vi "Initialize.vi"(8 "error in (no error)":errorcluster, 10 "DeviceName":string, 11 "HexapodController in":refnum<class "Tapedrive_ESP301.lvclass">) -> (0 "error out":errorcluster, 1 "new command(s)":string, 2 "DeviceName":string, 3 "HexapodController out":refnum<class "Tapedrive_ESP301.lvclass">)   [LabVIEW 2011, in "Tapedrive_ESP301.lvclass"]
uses:
  Tapedrive_ESP301.lvclass
  BaseDriver/BaseDriver.lvclass
  Tapedrive_ESP301.lvclass/Tapedrive_ESP301.ctl
  Newport ESP301.lvlib
panel:
  out "Cleared Error Queue":string
  out "Settings.devport":string
  out "Connected":bool
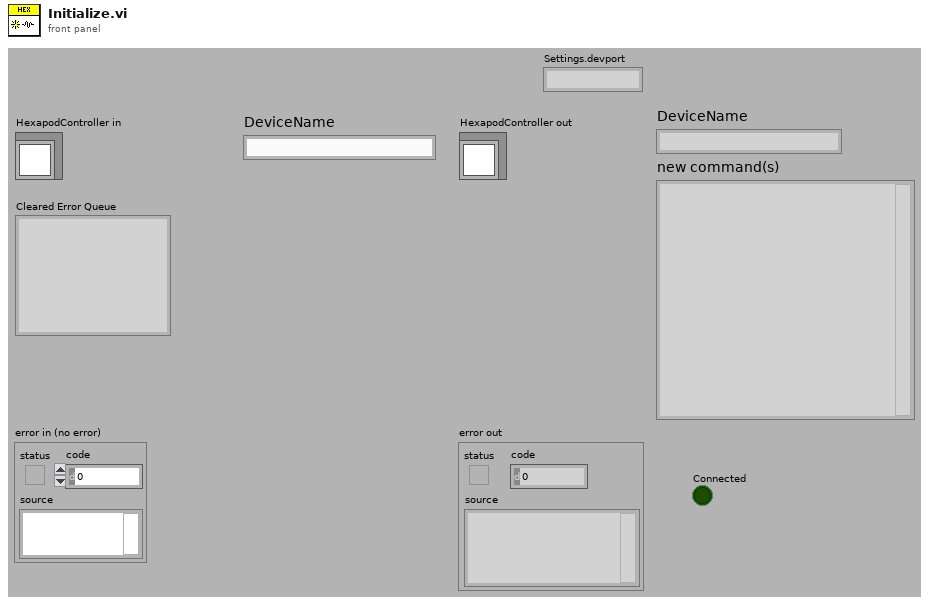
[diagram p1: front panel]
types:
  T1 = typedef "Tapedrive_ESP301.lvclass/settingsCluster_TapeDrive_TypDef.ctl" = cluster{"devport":string, "tapepos":cluster{"Value":dbl, "Min":dbl, "Max":dbl, "StepSize":dbl, "Tolerance":dbl, "ValueActual":dbl}, "status":enum16{"Not referenced", "Homing", "Moving", "Ready"}, "inmotion":T2, "forwardaxis":i16, "backwardaxis":i16, "encoderaxis":i16, "Velocity":cluster{"Axis 1":cluster{"Value":dbl, "Min":dbl, "Max":dbl, "StepSize":dbl, "Tolerance":dbl, "ValueActual":dbl}, "Axis 2":cluster{"Value":dbl, "Min":dbl, "Max":dbl, "StepSize":dbl, "Tolerance":dbl, "ValueActual":dbl}}, "Acceleration":cluster{"Axis 1":cluster{"Value":dbl, "Min":dbl, "Max":dbl, "StepSize":dbl, "Tolerance":dbl, "ValueActual":dbl}, "Axis 2":cluster{"Value":dbl, "Min":dbl, "Max":dbl, "StepSize":dbl, "Tolerance":dbl, "ValueActual":dbl}}, "Decceleration":cluster{"Axis 1":cluster{"Value":dbl, "Min":dbl, "Max":dbl, "StepSize":dbl, "Tolerance":dbl, "ValueActual":dbl}, "Axis 2":cluster{"Value":dbl, "Min":dbl, "Max":dbl, "StepSize":dbl, "Tolerance":dbl, "ValueActual":dbl}}, "MaxAcceleration":cluster{"Axis 1":cluster{"Value":dbl, "Min":dbl, "Max":dbl, "StepSize":dbl, "Tolerance":dbl, "ValueActual":dbl}, "Axis 2":cluster{"Value":dbl, "Min":dbl, "Max":dbl, "StepSize":dbl, "Tolerance":dbl, "ValueActual":dbl}}, "MaxVelocity":cluster{"Axis 1":cluster{"Value":dbl, "Min":dbl, "Max":dbl, "StepSize":dbl, "Tolerance":dbl, "ValueActual":dbl}, "Axis 2":cluster{"Value":dbl, "Min":dbl, "Max":dbl, "StepSize":dbl, "Tolerance":dbl, "ValueActual":dbl}}, "VelocityFFG":cluster{"Axis 1":cluster{"Value":dbl, "Min":dbl, "Max":dbl, "StepSize":dbl, "Tolerance":dbl, "ValueActual":dbl}, "Axis 2":cluster{"Value":dbl, "Min":dbl, "Max":dbl, "StepSize":dbl, "Tolerance":dbl, "ValueActual":dbl}}, "AccelerationFFG":cluster{"Axis 1":cluster{"Value":dbl, "Min":dbl, "Max":dbl, "StepSize":dbl, "Tolerance":dbl, "ValueActual":dbl}, "Axis 2":cluster{"Value":dbl, "Min":dbl, "Max":dbl, "StepSize":dbl, "Tolerance":dbl, "ValueActual":dbl}}, "DACoffset":cluster{"Axis 1":cluster{"Value":dbl, "Min":dbl, "Max":dbl, "StepSize":dbl, "Tolerance":dbl, "ValueActual":dbl}, "Axis 2":cluster{"Value":dbl, "Min":dbl, "Max":dbl, "StepSize":dbl, "Tolerance":dbl, "ValueActual":dbl}}, "Power":cluster{"Axis 1":T2, "Axis 2":T2}, "ReductionRatio":cluster{"Value":dbl, "Min":dbl, "Max":dbl, "StepSize":dbl, "Tolerance":dbl, "ValueActual":dbl}, "Direction":T3, "Tension":T2, "TensionVelocity":cluster{"Axis 1":cluster{"Value":dbl, "Min":dbl, "Max":dbl, "StepSize":dbl, "Tolerance":dbl, "ValueActual":dbl}, "Axis 2":cluster{"Value":dbl, "Min":dbl, "Max":dbl, "StepSize":dbl, "Tolerance":dbl, "ValueActual":dbl}}, "TensionAcceleration":cluster{"Axis 1":cluster{"Value":dbl, "Min":dbl, "Max":dbl, "StepSize":dbl, "Tolerance":dbl, "ValueActual":dbl}, "Axis 2":cluster{"Value":dbl, "Min":dbl, "Max":dbl, "StepSize":dbl, "Tolerance":dbl, "ValueActual":dbl}}, "TensionDecceleration":cluster{"Axis 1":cluster{"Value":dbl, "Min":dbl, "Max":dbl, "StepSize":dbl, "Tolerance":dbl, "ValueActual":dbl}, "Axis 2":cluster{"Value":dbl, "Min":dbl, "Max":dbl, "StepSize":dbl, "Tolerance":dbl, "ValueActual":dbl}}, "MoveVelocity":cluster{"Axis 1":cluster{"Value":dbl, "Min":dbl, "Max":dbl, "StepSize":dbl, "Tolerance":dbl, "ValueActual":dbl}, "Axis 2":cluster{"Value":dbl, "Min":dbl, "Max":dbl, "StepSize":dbl, "Tolerance":dbl, "ValueActual":dbl}}, "MoveAcceleration":cluster{"Axis 1":cluster{"Value":dbl, "Min":dbl, "Max":dbl, "StepSize":dbl, "Tolerance":dbl, "ValueActual":dbl}, "Axis 2":cluster{"Value":dbl, "Min":dbl, "Max":dbl, "StepSize":dbl, "Tolerance":dbl, "ValueActual":dbl}}, "MoveDecceleration":cluster{"Axis 1":cluster{"Value":dbl, "Min":dbl, "Max":dbl, "StepSize":dbl, "Tolerance":dbl, "ValueActual":dbl}, "Axis 2":cluster{"Value":dbl, "Min":dbl, "Max":dbl, "StepSize":dbl, "Tolerance":dbl, "ValueActual":dbl}}, "MaxStepsize":cluster{"Value":dbl, "Min":dbl, "Max":dbl, "StepSize":dbl, "Tolerance":dbl, "ValueActual":dbl}, "Stepsize":cluster{"Value":dbl, "Min":dbl, "Max":dbl, "StepSize":dbl, "Tolerance":dbl, "ValueActual":dbl}, "GoStep":T2, "StopWait":T2, "stepnum":cluster{"Value":dbl, "Min":dbl, "Max":dbl, "StepSize":dbl, "Tolerance":dbl, "ValueActual":dbl}, "MoveIfScan":T2, "HomeEncoder":T2, "Timeout":cluster{"Value":dbl, "Min":dbl, "Max":dbl, "StepSize":dbl, "Tolerance":dbl, "ValueActual":dbl}, "TapeRelax":cluster{"Value":dbl, "Min":dbl, "Max":dbl, "StepSize":dbl, "Tolerance":dbl, "ValueActual":dbl}}
  T2 = typedef "OnOffTypeDef.ctl" = enum16{"off", "on"}
  T3 = typedef "Direction.ctl" = enum16{"Forward", "Backward", "Undefined"}
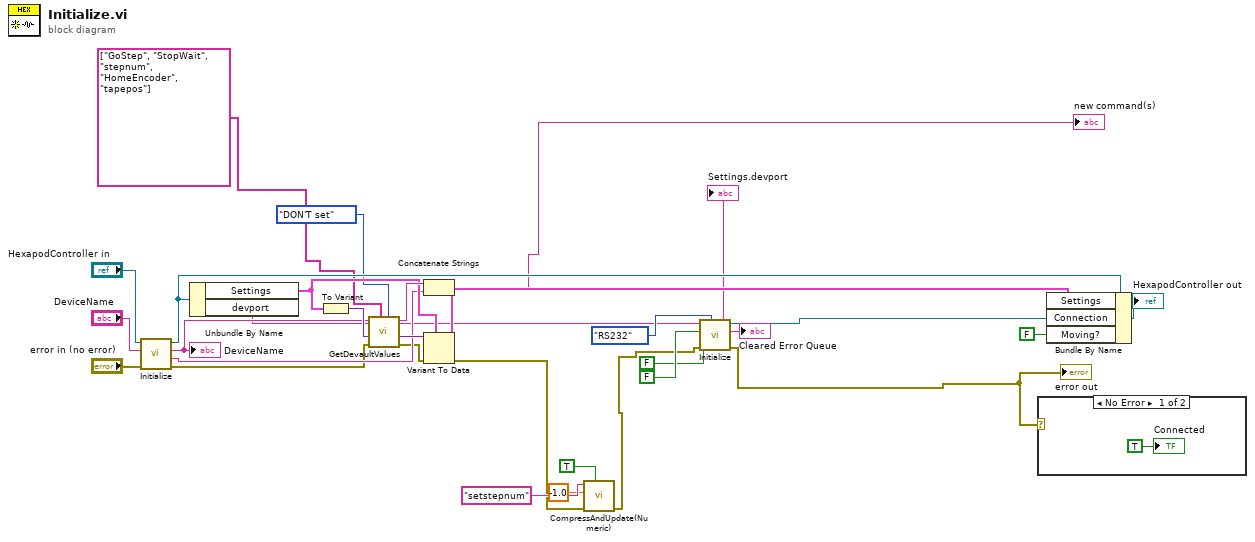
[diagram p0: block diagram]
diagram:
  n1 = call-parent "Initialize.vi"("error in (no error)"="error in (no error)", "DeviceName"="DeviceName", "BaseDriver in"="HexapodController in") -> ("error out"=w17:errorcluster, "new command(s)"=w22:string, "DeviceName"=w23:string, "BaseDriver out"=w21:refnum<class "Tapedrive_ESP301.lvclass">)  [unwired: 5 in]
  "DeviceName" <- w23
  n2 = Unbundle By Name(w21) -> ("Settings"=w24:T1, "devport"=w14:string)
  "Settings.devport" <- w14
  n3 = To Variant(anything=w24) -> (Variant=w25:variant)
  n4 = call "GetDevaultValues.vi"("set or DON'T set"=enum16{"set", "DON'T set"}."DON'T set", "set following Variables (empty = all avriables)"=string[] ["GoStep", "StopWait", "stepnum", "HomeEncoder", "tapepos"], "error in (no error)"=w17, "variant"=w25, "Device Name"=w23) -> ("error out"=w16:errorcluster, "variant out"=w26:variant, "new command(s)"=w27:string)  [unwired: 4 in]
  n5 = Concatenate Strings(w27, w22) -> (→"new command(s)":string)
  n6 = Variant To Data(error in=w16, type=w24, Variant=w26) -> (data=w19:T1, error out=w5:errorcluster)
  n7 = call "CompressAndUpdate(Numeric).vi"("force CVT update (false)"=TRUE, "error in"=w5, "Numeric"=-1.0, "command or variable name"="setstepnum") -> ("error out"=w4:errorcluster)  [unwired: 7 in]
  n8 = call "Initialize.vi"("VISA resource name"=w14, "ID Query (True)"=FALSE, "Reset (False)"=FALSE, "error in (no error)"=w4, "Serial Link (RS232)"=enum16{"RS232", "USB"}."RS232") -> ("VISA resource name out"=w3:refnum<visa-resource-name>, "Cleared Error Queue"=→"Cleared Error Queue":string, "error out"=w2:errorcluster)  [unwired: 3 in]
  "error out" <- w2
  n9 = case shown="No Error" w2 {
    frame No Error {
      "Connected" <- TRUE ("Connected")
    }
    frame Error {
    }
  }
  n10 = Bundle By Name(cluster=w21, "Settings"=w19, "Connection"=w3, "Moving?"=FALSE ("Wait for Step")) -> (→"HexapodController out":refnum<class "Tapedrive_ESP301.lvclass">)
